vi "Read Destination IP.vi"(8 "error in (no error)":errorcluster, 11 "TCP Writer in":refnum<class "TCP Writer.lvclass">) -> (0 "error out":errorcluster, 2 "Destination IP":string, 3 "TCP Writer out":refnum<class "TCP Writer.lvclass">)   [LabVIEW 2026, in "TALOS.lvlib" / "TCP Writer.lvlib" / "TCP Writer.lvclass"]
uses:
  TCP Writer.lvclass
  TCP Writer.lvclass/TCP Writer.ctl
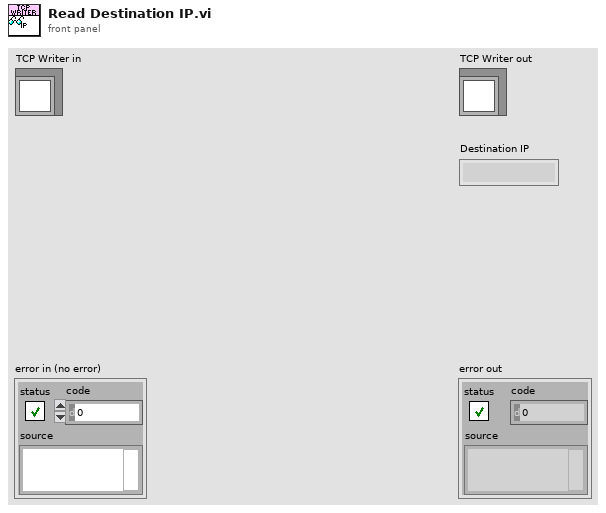
[diagram p1: front panel]
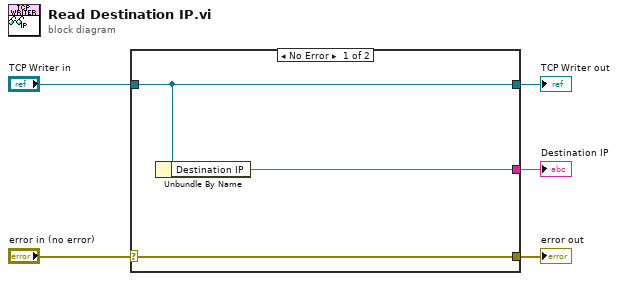
[diagram p0: block diagram]
diagram:
  n1 = case shown="No Error" "error in (no error)" {
    selector: "error in (no error)" -> [w8 w9]
    tunnel: [w8 w9] -> w4
    tunnel: [w7 w10] -> w2
    tunnel: "TCP Writer in" -> [w7 w10]
    tunnel: [w6 _] -> w1
    frame No Error {
      n2 = Unbundle By Name(w7) -> ("Destination IP"=w6:string)
    }
    frame Error {
    }
  }
  "error out" <- w4
  "TCP Writer out" <- w2
  "Destination IP" <- w1
